vi "runtest format quickmode key.vi"(1 "Quickmode Requested? (f)":bool, 2 "Any Quickmode Steps? (f)":bool, 3 "Allow Operator to Disable Quick Execution (f)":bool) -> (0 "QuickMode HTML":string)   [LabVIEW 2011]
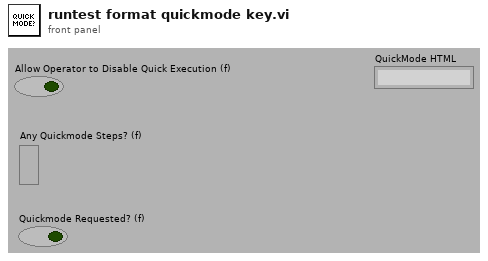
[diagram p1: front panel]
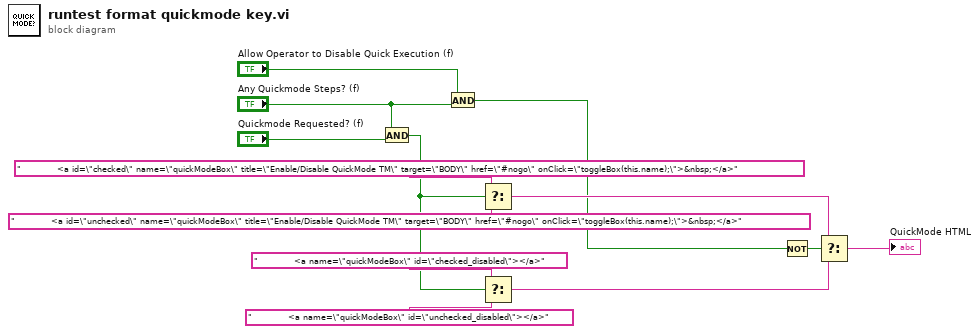
[diagram p0: block diagram]
diagram:
  n1 = And(x="Any Quickmode Steps? (f)", y="Quickmode Requested? (f)") -> (x .and. y?=w6:bool)
  n2 = And(x="Allow Operator to Disable Quick Execution (f)", y="Any Quickmode Steps? (f)") -> (x .and. y?=w5:bool)
  n3 = Select(t="            <a id=\"checked\" name=\"quickModeBox\" title=\"Enable/Disable QuickMode TM\" target=\"BODY\" href=\"#nogo\" onClick=\"toggleBox(this.name);\">&nbsp;</a>", s=w6, f="            <a id=\"unchecked\" name=\"quickModeBox\" title=\"Enable/Disable QuickMode TM\" target=\"BODY\" href=\"#nogo\" onClick=\"toggleBox(this.name);\">&nbsp;</a>") -> (s? t:f=w10:string)
  n4 = Select(t="            <a name=\"quickModeBox\" id=\"checked_disabled\"></a>", s=w6, f="            <a name=\"quickModeBox\" id=\"unchecked_disabled\"></a>") -> (s? t:f=w9:string)
  n5 = Not(x=w5) -> (.not. x?=w2:bool)
  n6 = Select(t=w10, s=w2, f=w9) -> (s? t:f=→"QuickMode HTML":string)
